vi "Gen Traj for Auto Pickup.vi"(0 "Path Positions":T1(array[cluster]), 1 "Robot Velocities":T2) -> (4 "Time & Dist":cluster{"Time (s)":dbl, "Distance (ft)":dbl}, 5 "Updated Waypoints":cluster{"x":dbl, "y":dbl, "th":dbl}[](array[cluster]), 6 "Trajectory Data Out":T5(array[cluster]))   [LabVIEW 2025]
uses:
  bordeaux/Bordeaux/Types/Segment Type.ctl
  bordeaux/Bordeaux/Types/Limits.ctl
  swerve-template/Type Definitions/Data/Robot Velocities.ctl
  bordeaux/Bordeaux/Types/Angluar Limits.ctl
  bordeaux/Bordeaux/Types/Drive Type.ctl
panel:
  out "Velocity Waveform":dbl[](graph)=[7.294446746788231, 7.794446746788231, 8.294446746788232, 8.794446746788232, 9.294446746788232, 9.794446746788232, 9.794446746788232, 9.794446746788232, 9.794446746788232, 9.294446746788232, 8.794446746788232, 8.294446746788232, 7.794446746788232, 7.294446746788232, 6.794446746788232, 6.294446746788232, 5.794446746788232, 5.294446746788232, 4.794446746788232, 4.294446746788232, 3.794446746788232, 3.294446746788232, 2.794446746788232, 2.294446746788232, 1.794446746788232, 1.294446746788232, 0.7944467467882319, 0.2944467467882319, 0.0]
  in  "Limits":T3={"Velocity (fps)"=10.0, "Accel (fps^2)"=22.0, "Jerk (fps^3)"=4000.0, "StoopidFast (fps)"=10.0} {"StoopidFast (fps)" min=0.0; "Jerk (fps^3)" min=0.0 step=1.0; "Accel (fps^2)" min=0.0; "Velocity (fps)" min=0.0}
  out "Past Generation Speed":u32
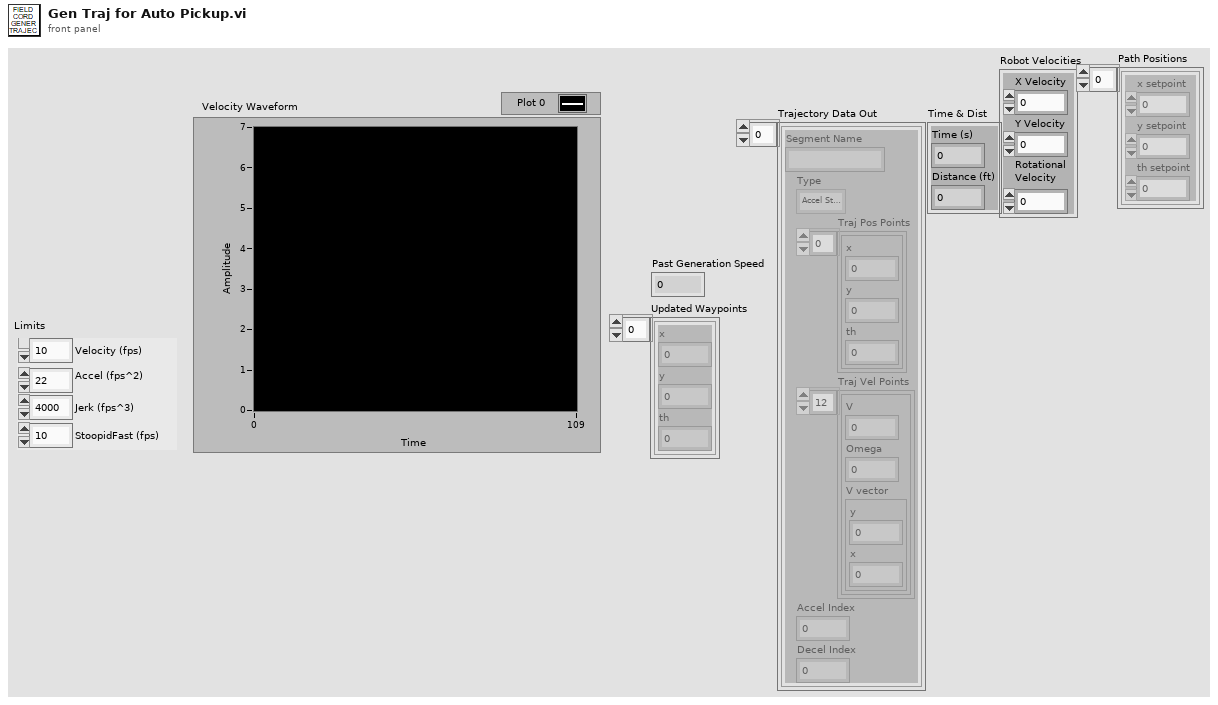
[diagram p1: front panel]
types:
  T1 = cluster{"x setpoint":dbl, "y setpoint":dbl, "th setpoint":dbl}[]
  T2 = typedef "Robot Velocities.ctl" = cluster{"X Velocity":dbl, "Y Velocity":dbl, "Rotational \nVelocity":dbl}
  T3 = typedef "Limits.ctl" = cluster{"Velocity (fps)":dbl, "Accel (fps^2)":dbl, "Jerk (fps^3)":dbl, "StoopidFast (fps)":dbl}
  T4 = typedef "Segment Type.ctl" = enum16{"Accel Straight", "Const Straight", "Blend", "Circle", "Bezier"}
  T5 = cluster{"Segment Name":string, "Type":T4, "Traj Pos Points":cluster{"x":dbl, "y":dbl, "th":dbl}[], "Traj Vel Points":cluster{"V":dbl, "Omega":dbl, "V vector":cluster{"y":dbl, "x":dbl}}[], "Accel Index":i32, "Decel Index":i32}[]
  T6 = typedef "Drive Type.ctl" = enum16{"Nonholonomic", "Holonomic"}
  T7 = typedef "Angluar Limits.ctl" = cluster{"Velocity (deg/s)":dbl, "Accel (deg/s^2)":dbl, "Jerk (deg/s^3)":dbl}
  T8 = cluster{"V":dbl, "Omega":dbl, "V vector":cluster{"y":dbl, "x":dbl}}[]
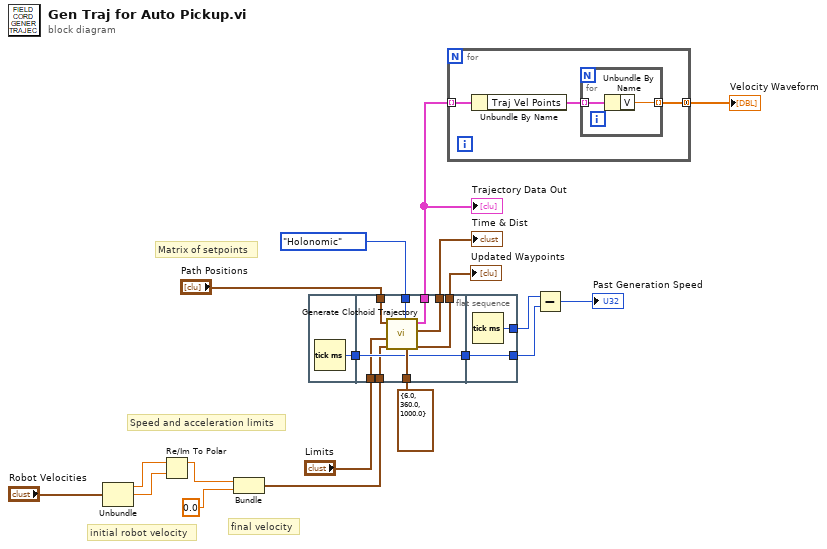
[diagram p0: block diagram]
diagram:
  # "initial robot velocity"
  # "Speed and acceleration limits"
  # "Matrix of setpoints"
  # "final velocity"
  n1 = Unbundle("Robot Velocities") -> ("X Velocity"=w19:dbl, "Y Velocity"=w18:dbl)  [unwired: 1 out]
  n2 = Re/Im To Polar(2:w18, 3:w19) -> (1:w13:dbl)  [unwired: 1 out]
  n3 = Bundle(w13, 0.0) -> (w7:cluster{dbl, dbl})  [unwired: 1 in]
  n4 = flat-sequence {
    tunnel: [w20] -> w17
    tunnel: Drive_Type."Holonomic" ("Drive Type") -> [w29]
    tunnel: T7 {"Velocity (deg/s)"=6.0, "Accel (deg/s^2)"=360.0, "Jerk (deg/s^3)"=1000.0} ("Angular Limits") -> [w28]
    tunnel: [w27] -> w4
    tunnel: w17 -> [w26]
    tunnel: [w26] -> w16
    tunnel: [w25] -> w11
    tunnel: [w24] -> w3
    tunnel: "Path Positions" -> [w23]
    tunnel: w7 -> [w22]
    tunnel: "Limits" -> [w21]
    tunnel: [w31] -> w10
    tunnel: w16 -> [w30]
    tunnel: [w30] -> w9
    frame #0 {
      n5 = Tick Count (ms)() -> (millisecond timer value=w20:u32)
    }
    frame #1 {
      n6 = call "Generate Clothoid Trajectory.vi"("Angular Limits"=w28, "Drive Type"=w29, "Conditions"=w22, "Limits"=w21, "WayPoints"=w23) -> ("Updated Waypoints"=w24:cluster{"x":dbl, "y":dbl, "th":dbl}[], "Time & Dist"=w25:cluster{"Time (s)":dbl, "Distance (ft)":dbl}, "Trajectory Data Out"=w27:T5)  [unwired: 3 in, 1 out]
    }
    frame #2 {
      n7 = Tick Count (ms)() -> (millisecond timer value=w31:u32)
    }
  }
  n8 = for {
    tunnel: [w33] -> w5 mode=concatenating
    tunnel: w4 -> [w32] mode=indexing
    n9 = Unbundle By Name(w32) -> ("Traj Vel Points"=w34:T8)
    n10 = for {
      tunnel: w34 -> [w36] mode=indexing
      tunnel: [w35] -> w33 mode=indexing
      n11 = Unbundle By Name(w36) -> ("V"=w35:dbl)
    }
  }
  "Velocity Waveform" <- w5
  n12 = Subtract(x=w10, y=w9) -> (x-y=→"Past Generation Speed":u32)
  "Trajectory Data Out" <- w4
  "Time & Dist" <- w11
  "Updated Waypoints" <- w3
